vi "corridor_math.vi"(6 "Corridor Width":dbl, 8 "Waypoint Y":dbl, 9 "Waypoint X":dbl, 10 "Irons Range":dbl, 11 "Boat Angle":dbl(slide) scale=0.0..360.0) -> (0 "Y out":dbl, 1 "X out":dbl)   [LabVIEW 2013]
doc: "Tacking math with corridor-shaped boundaries implemented.\n\n23 Jan. 2015\nJoe Sutker"
panel:
  in  "min tack length":dbl
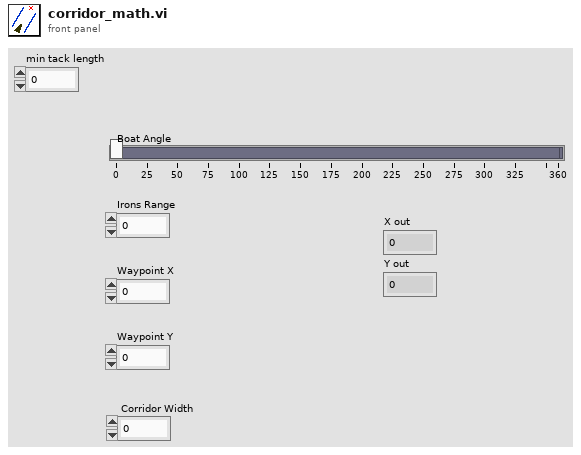
[diagram p1: front panel]
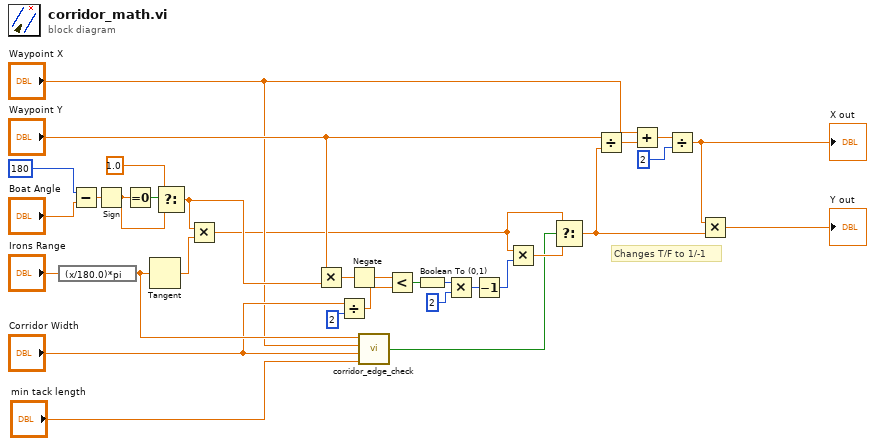
[diagram p0: block diagram]
diagram:
  # "Changes T/F to 1/-1"
  n1 = expression code="(x/180.0)*pi"("Irons Range") -> (w7:dbl)
  n2 = Subtract(x=180, y="Boat Angle") -> (x-y=w32:dbl)
  n3 = Sign(1:w32) -> (0:w29:dbl)
  n4 = Equal To 0?(x=w29) -> (x = 0?=w31:bool)
  n5 = Tangent(1:w7) -> (0:w28:dbl)
  n6 = Select(t=1.0, s=w31, f=w29) -> (s? t:f=w17:dbl)
  n7 = Multiply(x=w17, y=w28) -> (x*y=w4:dbl)
  n8 = Multiply(x="Waypoint Y", y=w17) -> (x*y=w16:dbl)
  n9 = Divide(x="Corridor Width", y=2) -> (x/y=w19:dbl)
  n10 = Negate(x=w16) -> (-x=w15:dbl)
  n11 = call "corridor_edge_check.vi"("min tack length"="min tack length", "corridor width"="Corridor Width", "Waypoint X Coordinate"="Waypoint X", "angle"=w7) -> ("Out of Corridor"=w8:bool)
  n12 = Less?(x=w15, y=w19) -> (x < y?=w14:bool)
  n13 = Boolean To (0,1)(Boolean=w14) -> (0, 1=w13:i16)
  n14 = Multiply(x=w13, y=2) -> (x*y=w11:i32)
  n15 = Decrement(x=w11) -> (x-1=w10:i32)
  n16 = Multiply(x=w4, y=w10) -> (x*y=w9:dbl)
  n17 = Select(t=w4, s=w8, f=w9) -> (s? t:f=w3:dbl)
  n18 = Divide(x="Waypoint Y", y=w3) -> (x/y=w27:dbl)
  n19 = Add(x="Waypoint X", y=w27) -> (x+y=w26:dbl)
  n20 = Divide(x=w26, y=2) -> (x/y=w22:dbl)
  "X out" <- w22
  n21 = Multiply(x=w22, y=w3) -> (x*y=→"Y out":dbl)
